vi "Periodic Tasks.vi"(8 "error in":errorcluster) -> ()   [LabVIEW 2012]
doc: "This VI runs in parallel to other tasks. It can contain as many user-defined periodic loops as you need. These can carry out PID or other sorts of timed response."
uses:
  <vilib>/Rock Robotics/SystemInterfaces/Utilities/FPGA_UtilitiesLED Source.ctl
  <vilib>/Rock Robotics/SystemInterfaces/Utilities/FPGA_UtilitiesLED State.ctl
  <vilib>/Rock Robotics/WPI/Relay/WPI_RelayValue.ctl
  <vilib>/Rock Robotics/WPI/Solenoid/WPI_SolenoidValue.ctl
  <vilib>/Rock Robotics/WPI/DriverStation/DriverStationLCD/WPI_DriverStationLCDLCDLine.ctl
  <vilib>/Rock Robotics/WPI/SafetyOutput/WPI_SafetyOutputConfigMenu.ctl
  Begin/Global Refnums.vi
  Begin/Global Variables.vi
  <vilib>/Rock Robotics/WPI/Solenoid/WPI_SolenoidSetEnum.vi
  <vilib>/Rock Robotics/WPI/Compressor/WPI_CompressorGetSetRefNum.vi
  Begin/Robot Global Data.vi
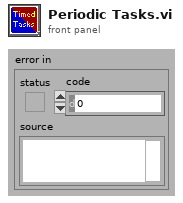
[diagram p1: front panel]
types:
  T1 = typedef "WPI_SolenoidValue.ctl" = enum16{"Off", "On", "Forward", "Reverse"}
  T2 = typedef "WPI_SafetyOutputConfigMenu.ctl" = enum16{"Enable", "Disable"}
  T3 = typedef "WPI_DriverStationLCDLCDLine.ctl" = enum16{"Main - Line 1", "User - Line 2", "User - Line 3", "User - Line 4", "User - Line 5", "User - Line 6"}
  T4 = typedef "WPI_SolenoidDevRef.ctl" = cluster{"DevStatus":errorcluster, "Solenoid Module":T5, "Forward Solenoid Channel":T6, "Reverse Solenoid Channel":T6}
  T5 = typedef "FPGA_TypedefSolenoidModule.ctl" = enum16{"Solenoid Module 1", "Solenoid Module 2"}
  T6 = typedef "WPI_SolenoidChannel.ctl" = enum8{"Solenoid 1", "Solenoid 2", "Solenoid 3", "Solenoid 4", "Solenoid 5", "Solenoid 6", "Solenoid 7", "Solenoid 8", "Invalid"}
  T7 = typedef "WPI_MotorControlDeviceRef.ctl" = cluster{"DeviceStatus":errorcluster, "Type":enum16{"PWM", "CAN"}, "PWM":cluster{"Digital Module":T8, "PWM Channel":T9, "DeadBand":T10}, "CAN":cluster{"Device Number":u8, "Control Mode":T11, "Semaphore":T12, "Max Vout":dbl}, "Invert":bool, "TransformRef":T13, "InvTransformRef":T13}
  T8 = typedef "FPGA_TypedefDigitalModule.ctl" = enum16{"Digital Module 1", "Digital Module 2"}
  T9 = typedef "FPGA_DIOPWMChannel.ctl" = enum8{"PWM 1", "PWM 2", "PWM 3", "PWM 4", "PWM 5", "PWM 6", "PWM 7", "PWM 8", "PWM 9", "PWM 10", "Invalid"}
  T10 = typedef "WPI_PWMDeadband.ctl" = cluster{"Name":string, "maxPositivePwm":i32, "minPositivePwm":i32, "centerPwm":i32, "maxNegativePwm":i32, "minNegativePwm":i32, "angularRange":u16}
  T11 = typedef "WPI_CANJaguar_ControlMode.ctl" = enum8{"Percent VBus", "Current", "Speed", "Position", "Voltage"}
  T12 = typedef "Semaphore RefNum" = refnum<k1>
  T13 = typedef "WPI_PWMTransform_ConPane.ctl" = refnum<vi>
  T14 = typedef "FPGA_UtilitiesLED State.ctl" = enum16{"Off", "On", "Toggle"}
  T15 = typedef "FPGA_UtilitiesLED Source.ctl" = enum16{"User LED", "FPGA LED"}
  T16 = typedef "WPI_RelayValue.ctl" = enum16{"Off", "On", "Forward", "Reverse"}
  T17 = typedef "WPI_CompressorDevRef.ctl" = cluster{"DevStatus":errorcluster, "DigitalInputDevRef":T18, "RelayDevRef":T20}
  T18 = typedef "WPI_DigitalInputDevRef.ctl" = cluster{"DevStatus":errorcluster, "DIO Channel":T19, "Digital Module":T8}
  T19 = typedef "FPGA_DIOChannel.ctl" = enum8{"DIO 1", "DIO 2", "DIO 3", "DIO 4", "DIO 5", "DIO 6", "DIO 7", "DIO 8", "DIO 9", "DIO 10", "DIO 11", "DIO 12", "DIO 13", "DIO 14", "Invalid"}
  T20 = typedef "WPI_RelayDevRef.ctl" = cluster{"DevStatus":errorcluster, "Relay Channel":T21, "Digital Module":T8, "Relay Direction":T22}
  T21 = typedef "FPGA_DIORelayChannel.ctl" = enum8{"Relay 1", "Relay 2", "Relay 3", "Relay 4", "Relay 5", "Relay 6", "Relay 7", "Relay 8", "Invalid"}
  T22 = typedef "WPI_RelayDirection.ctl" = enum16{"Both directions", "Forward only", "Reverse only"}
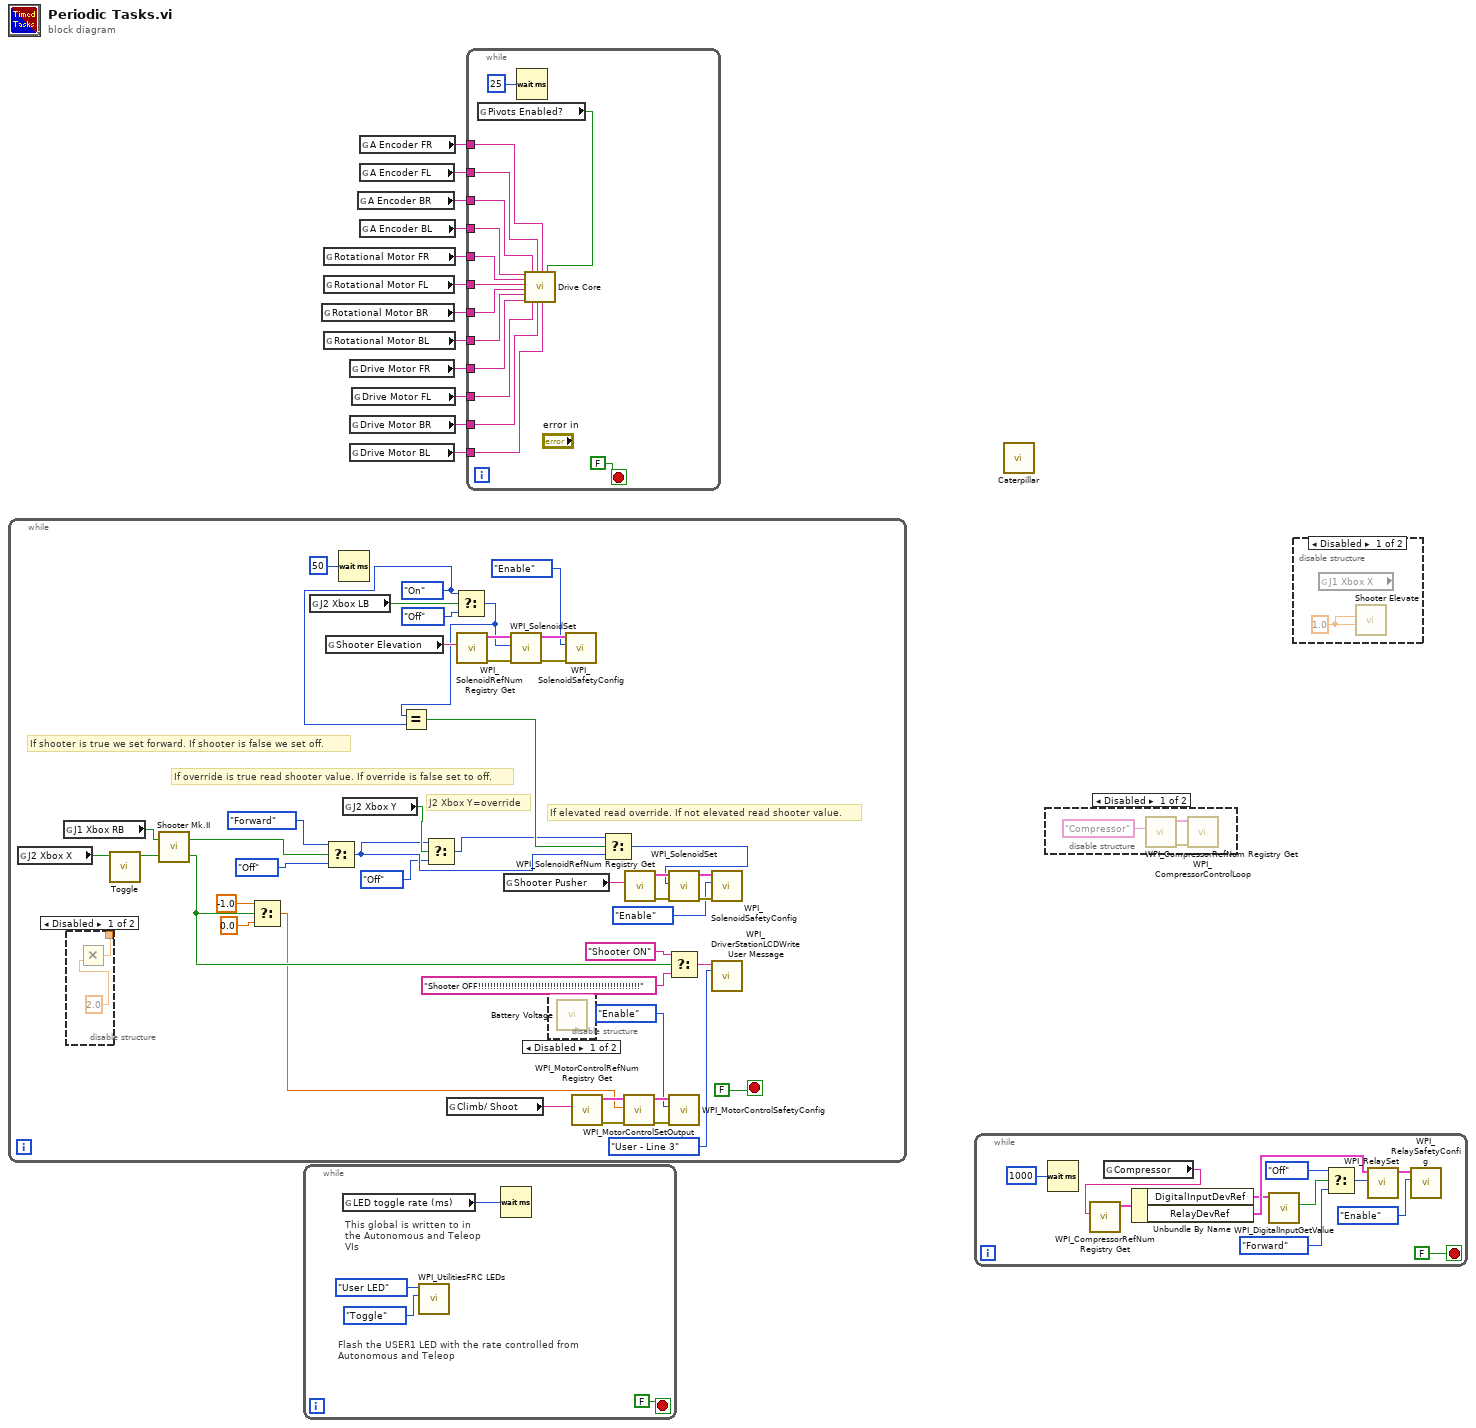
[diagram p0: block diagram]
diagram:
  n1 = while {
    stop <- FALSE stop-if-true
    w21 = WPI_SolenoidValue."On" ("Value")
    # "J2 Xbox Y=override"
    # "If elevated read override. If not elevated read shooter value."
    # "If override is true read shooter value. If override is false set to off."
    # "If shooter is true we set forward. If shooter is false we set off."
    n2 = global read "Global Variables.vi" "J2 Xbox X"() -> (w41:bool)
    n3 = global read "Global Variables.vi" "J1 Xbox RB"() -> (w30:bool)
    n4 = disable-structure shown="Disabled" {
      disable-tunnel: [w58 _] -> _
      frame Disabled {
        n5 = Multiply(y=2.0) -> (x*y=w58:dbl)  [unwired: 1 in]
      }
      frame Enabled {
      }
    }
    n6 = call "Toggle.vi"("Boolean"=w41) -> ("Toggled"=w31:bool)  [unwired: 10 in]
    n7 = call "Shooter Mk.II.vi"("Motor"=w31, "Fire"=w30) -> ("Shooter On"=w23:bool, "Extend Shooter"=w33:bool)
    n8 = Select(t=-1.0, s=w23, f=0.0) -> (s? t:f=w14:dbl)
    n9 = global read "Global Variables.vi" "J2 Xbox LB"() -> (w39:bool)
    n10 = global read "Global Refnums.vi" "Shooter Elevation"() -> (w44:string)
    n11 = Select(t=WPI_SolenoidValue."Forward", s=w33, f=WPI_SolenoidValue."Off" ("Value")) -> (s? t:f=w17:T1)
    n12 = Wait (ms)(milliseconds to wait=u32 50) -> ()  [unwired: 1 out]
    n13 = global read "Global Variables.vi" "J2 Xbox Y"() -> (w18:bool)
    n14 = Select(t=w17, s=w18, f=WPI_SolenoidValue."Off" ("Value")) -> (s? t:f=w16:T1)
    n15 = global read "Global Refnums.vi" "Climb/ Shoot"() -> (w24:string)
    n16 = Select(t=w21, s=w39, f=WPI_SolenoidValue."Off" ("Value")) -> (s? t:f=w22:T1)
    n17 = Equal?(x=w22, y=w21) -> (x = y?=w20:bool)
    n18 = call <vilib>:"WPI_SolenoidRefNum Registry Get.vi"("refnum name"=w44) -> ("error out"=w48:errorcluster, "SolenoidDevRef"=w49:T4)  [unwired: 9 in]
    n19 = global read "Global Refnums.vi" "Shooter Pusher"() -> (w43:string)
    n20 = call-poly <vilib>:"WPI_SolenoidSet.vi"("error in (no error)"=w48, "Value"=w22, "SolenoidDevRef"=w49) -> ("error out"=w46:errorcluster, "SolenoidDevRef"=w47:T4)  [unwired: 7 in]
    n21 = disable-structure shown="Disabled" {
      frame Disabled {
        n22 = call "Battery Voltage.vi"() -> ()  [unwired: 1 out]
      }
      frame Enabled {
      }
    }
    n23 = call <vilib>:"WPI_SolenoidSafetyConfig.vi"("error in (no error)"=w46, "mode"=WPI_SafetyOutputConfigMenu."Enable", "SolenoidDevRef"=w47) -> ()  [unwired: 7 in, 2 out]
    n24 = call <vilib>:"WPI_MotorControlRefNum Registry Get.vi"("refnum name"=w24) -> ("error out"=w28:errorcluster, "MotorControlDevRef"=w29:T7)  [unwired: 9 in]
    n25 = Select(t=w16, s=w20, f=w17) -> (s? t:f=w19:T1)
    n26 = call <vilib>:"WPI_MotorControlSetOutput.vi"("error in (no error)"=w28, "Output"=w14, "MotorControlDevRef"=w29) -> ("error out"=w26:errorcluster, "MotorControlDevRef"=w27:T7)  [unwired: 6 in, 1 out]
    n27 = call <vilib>:"WPI_SolenoidRefNum Registry Get.vi"("refnum name"=w43) -> ("error out"=w55:errorcluster, "SolenoidDevRef"=w56:T4)  [unwired: 9 in]
    n28 = call-poly <vilib>:"WPI_SolenoidSet.vi"("error in (no error)"=w55, "Value"=w19, "SolenoidDevRef"=w56) -> ("error out"=w54:errorcluster, "SolenoidDevRef"=w53:T4)  [unwired: 7 in]
    n29 = Select(t="Shooter ON", s=w23, f="Shooter OFF!!!!!!!!!!!!!!!!!!!!!!!!!!!!!!!!!!!!!!!!!!!!!!!!!!!!!!") -> (s? t:f=w35:string)
    n30 = call <vilib>:"WPI_MotorControlSafetyConfig.vi"("error in (no error)"=w26, "mode"=WPI_SafetyOutputConfigMenu."Enable", "MotorControlDevRef"=w27) -> ()  [unwired: 7 in, 2 out]
    n31 = call <vilib>:"WPI_SolenoidSafetyConfig.vi"("error in (no error)"=w54, "mode"=WPI_SafetyOutputConfigMenu."Enable", "SolenoidDevRef"=w53) -> ()  [unwired: 7 in, 2 out]
    n32 = call <vilib>:"WPI_DriverStationLCDWrite User Message.vi"("line text"=w35, "line"=WPI_DriverStationLCDLCDLine."User - Line 3") -> ()  [unwired: 13 in, 1 out]
  }
  n33 = while {
    stop <- FALSE stop-if-true
    # "This global is written to in the Autonomous and Teleop VIs"
    # "Flash the USER1 LED with the rate controlled from Autonomous and Teleop"
    n34 = global read "Robot Global Data.vi" "LED toggle rate (ms)"() -> (w59:u32)
    n35 = call <vilib>:"WPI_UtilitiesFRC LEDs.vi"("State"=FPGA_UtilitiesLED_State."Toggle", "LED Type"=FPGA_UtilitiesLED_Source."User LED") -> ()  [unwired: 1 in, 9 out]
    n36 = Wait (ms)(milliseconds to wait=w59) -> ()  [unwired: 1 out]
  }
  n37 = global read "Global Refnums.vi" "Rotational Motor BR"() -> (w3:string)
  n38 = global read "Global Refnums.vi" "Rotational Motor FR"() -> (w4:string)
  n39 = global read "Global Refnums.vi" "Rotational Motor FL"() -> (w1:string)
  n40 = global read "Global Refnums.vi" "Rotational Motor BL"() -> (w2:string)
  n41 = global read "Global Refnums.vi" "Drive Motor FR"() -> (w8:string)
  n42 = global read "Global Refnums.vi" "Drive Motor BR"() -> (w7:string)
  n43 = global read "Global Refnums.vi" "Drive Motor BL"() -> (w6:string)
  n44 = global read "Global Refnums.vi" "Drive Motor FL"() -> (w5:string)
  n45 = global read "Global Refnums.vi" "A Encoder BR"() -> (w11:string)
  n46 = global read "Global Refnums.vi" "A Encoder FR"() -> (w12:string)
  n47 = global read "Global Refnums.vi" "A Encoder FL"() -> (w9:string)
  n48 = global read "Global Refnums.vi" "A Encoder BL"() -> (w10:string)
  n49 = while {
    tunnel: w12 -> [w76]
    tunnel: w11 -> [w74]
    tunnel: w10 -> [w73]
    tunnel: w9 -> [w75]
    tunnel: w8 -> [w68]
    tunnel: w7 -> [w66]
    tunnel: w6 -> [w65]
    tunnel: w5 -> [w67]
    tunnel: w4 -> [w72]
    tunnel: w3 -> [w70]
    tunnel: w2 -> [w69]
    tunnel: w1 -> [w71]
    stop <- FALSE stop-if-true
    n50 = global read "Global Variables.vi" "Pivots Enabled?"() -> (w63:bool)
    n51 = Wait (ms)(milliseconds to wait=u32 25) -> ()  [unwired: 1 out]
    n52 = call "Drive Core.vi"("A Encoder BL"=w73, "Rotational Motor FR"=w72, "Rotational Motor FL"=w71, "Rotational Motor BR"=w70, "Rotational Motor BL"=w69, "Drive Motor FR"=w68, "A Encoder BR"=w74, "Drive Motor FL"=w67, "A Encoder FL"=w75, "Drive Motor BR"=w66, "A Encoder FR"=w76, "Drive Motor BL"=w65, "Enabled?"=w63) -> ()  [unwired: 7 in]
  }
  n53 = while {
    stop <- FALSE stop-if-true
    n54 = Wait (ms)(milliseconds to wait=u32 1000) -> ()  [unwired: 1 out]
    n55 = global read "Global Refnums.vi" "Compressor"() -> (w78:string)
    n56 = call <vilib>:"WPI_CompressorRefNum Registry Get.vi"("refnum name"=w78) -> ("CompressorDevRef"=w89:T17)  [unwired: 9 in, 1 out]
    n57 = Unbundle By Name(w89) -> ("DigitalInputDevRef"=w87:T18, "RelayDevRef"=w88:T20)
    n58 = call <vilib>:"WPI_DigitalInputGetValue.vi"("DigitalInputDevRef"=w87) -> ("Value"=w86:bool)  [unwired: 8 in, 2 out]
    n59 = Select(t=WPI_RelayValue."Off" ("RelayValue"), s=w86, f=WPI_RelayValue."Forward" ("RelayValue")) -> (s? t:f=w81:T16)
    n60 = call <vilib>:"WPI_RelaySet.vi"("RelayValue"=w81, "RelayDevRef"=w88) -> ("RelayDevRef"=w83:T20)  [unwired: 8 in, 1 out]
    n61 = call <vilib>:"WPI_RelaySafetyConfig.vi"("mode"=WPI_SafetyOutputConfigMenu."Enable", "RelayDevRef"=w83) -> ()  [unwired: 8 in, 2 out]
  }
  n62 = call "Caterpillar.vi"() -> ()  [unwired: 12 in]
  n63 = disable-structure shown="Disabled" {
    frame Disabled {
      n64 = call <vilib>:"WPI_CompressorRefNum Registry Get.vi"("refnum name"="Compressor") -> ("error out"=w92:errorcluster, "CompressorDevRef"=w91:T17)  [unwired: 9 in]
      n65 = call <vilib>:"WPI_CompressorControlLoop.vi"("error in (no error)"=w92, "CompressorDevRef"=w91) -> ()  [unwired: 10 in]
    }
    frame Enabled {
    }
  }
  n66 = disable-structure shown="Disabled" {
    frame Disabled {
      w93 = 1.0 ("Lowering time (s)")
      n67 = global read "Global Variables.vi" "J1 Xbox X"() -> ()  [unwired: 1 out]
      n68 = call "Shooter Elevate.vi"("Elevation time (s)"=w93, "Lowering time (s)"=w93) -> ()  [unwired: 8 in, 2 out]
    }
    frame Enabled {
    }
  }
